vi "WiFi lab coordinator API.vi"() -> ()   [LabVIEW 2021]
uses:
  WiFi API Frame Type.ctl
  WiFi API Frame.ctl
  stop button.vi
  <vilib>/Utility/file.llb/Write Delimited Spreadsheet (string).vi
panel:
  in  "Response TCP":string
  in  "stop":bool
  in  "Response UDP":string
  in  "Control string":string
  in  "Start session":bool
  in  "Destination port (hex)":u16=9750 step=1 format="%04x"
  in  "Source port (hex)":u16=2000 step=1 format="%04x"
  out "IPs":T1(array[cluster])
  out "Payload":string
  out "Frame Type":T2 items=["Frame Error"=254, "Device Response Status"=186, "Device Request"=185, "Send Data Response"=184, "RX Packet IPv4"=176, "Zigbee Remote AT Command Response"=151, "Explicit Zigbee Receive Packet"=145, "Zigbee Receive Packet"=144, "I/O Sample Rx Indicator"=143, "Zigbee TX Status"=139, "Modem Status"=138, "Transmit Status"=137, "AT Command Response"=136, "Remote Command Response"=135, "Rx Packet"=128, "Device Response"=42, "Send Data Request"=40, "TX Request IPv4"=32, "Zigbee Remote AT Command"=23, "Zigbee Explicit Transmit Packet"=17, "Zigbee Transmit Packet"=16, "AT Command "=8, "Remote AT Command Request"=7, "TX Request"=0]
  # "Session Configuration"
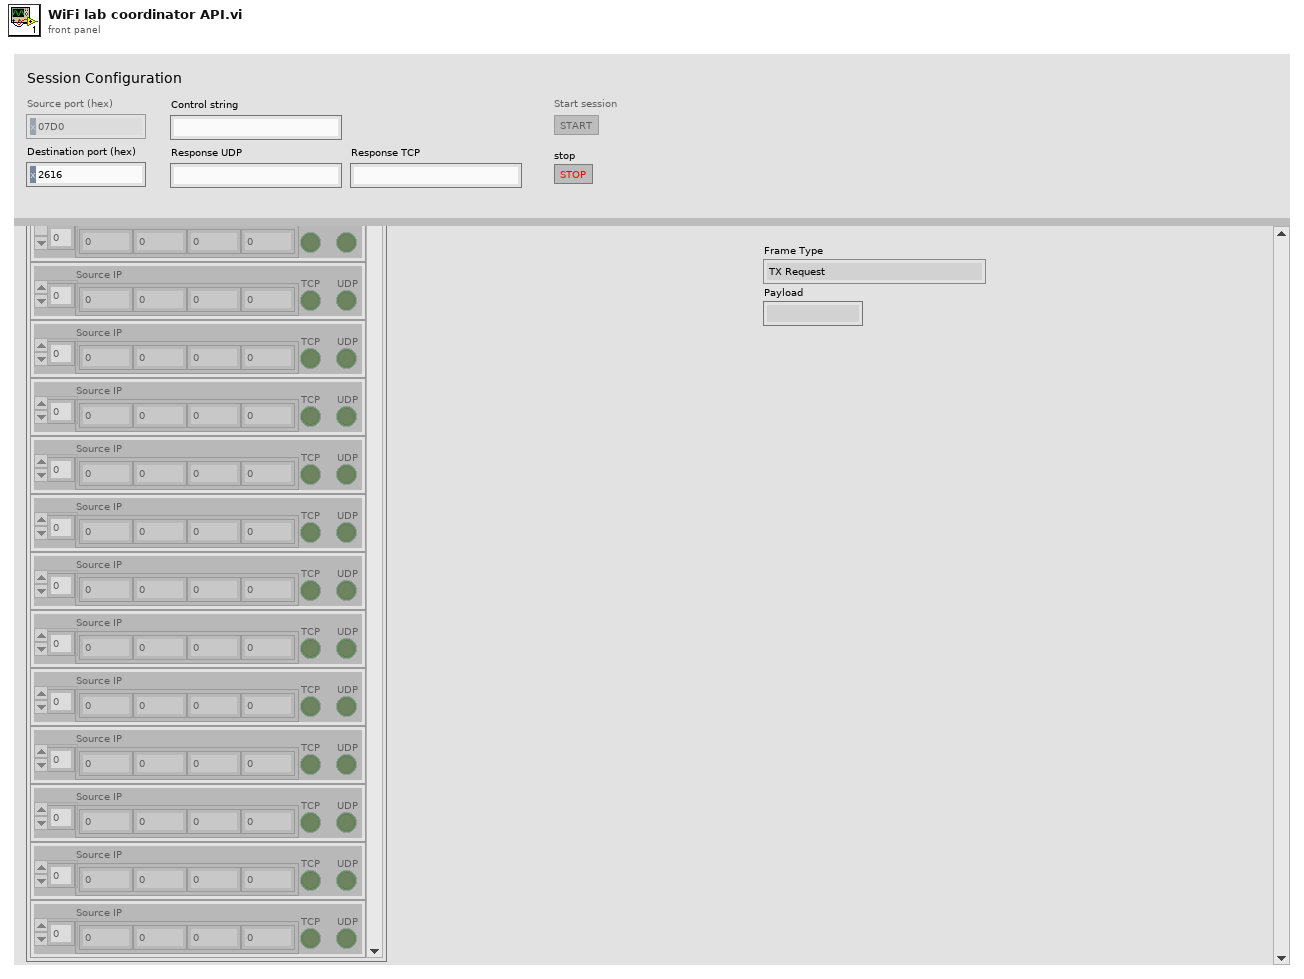
[diagram p1: front panel]
types:
  T1 = cluster{"Source IP":u8[], "TCP":bool, "UDP":bool}[]
  T2 = typedef "WiFi API Frame Type.ctl" = u8
  T3 = cluster{"Source IP":u8[], "TCP":bool, "UDP":bool}
  T4 = typedef "WiFi API Frame.ctl" = cluster{"Length":u16, "Frame Type":T2, "Payload":u8[], "Checksum":u8}
  T5 = enum8{"Enabled", "Disabled", "Disabled and Grayed Out"}
  T6 = typedef "Protocol enum.ctl" = enum8{"UDP", "TCP"}
  T7 = enum32{"invalid app kind", "Development System", "Run Time System", "Student Edition", "Embedded LabVIEW", "Evaluation", "Custom"}
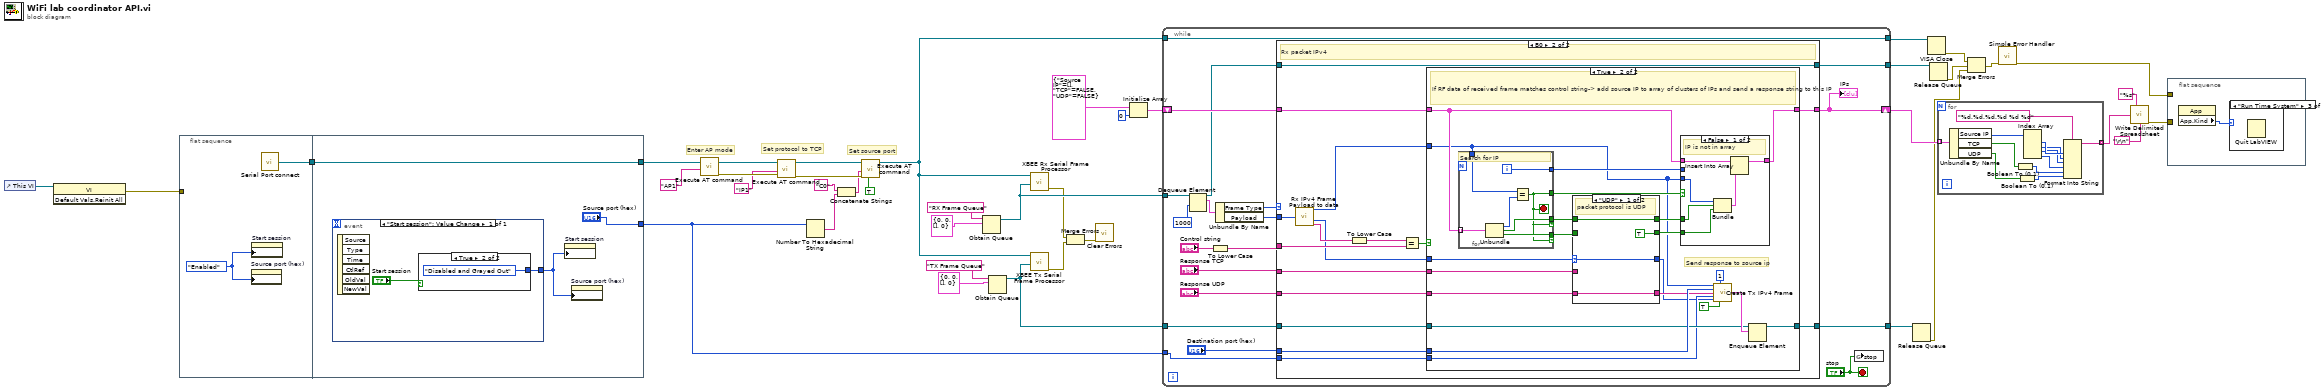
[diagram p0: block diagram]
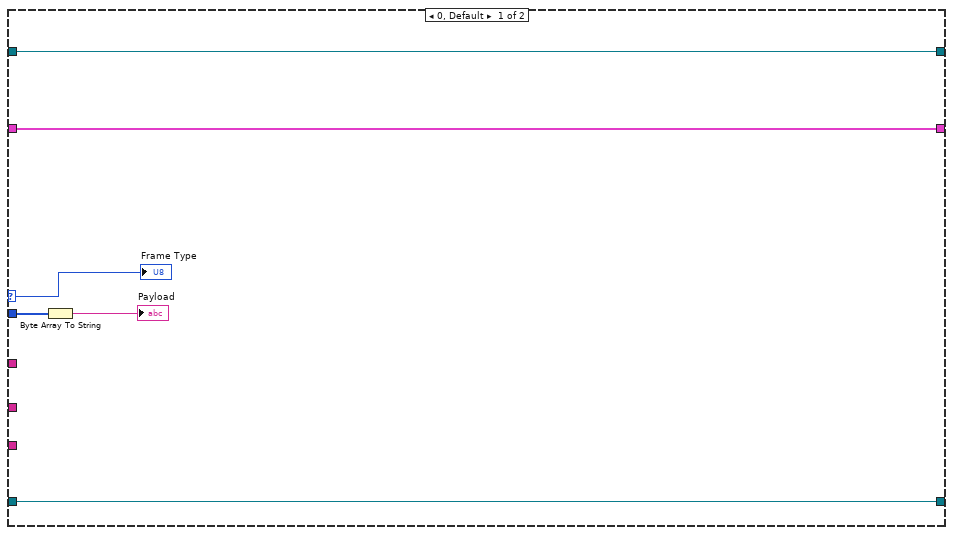
[diagram p8: hidden frame]
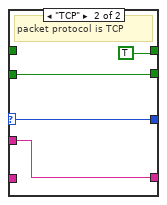
[diagram p10: hidden frame]
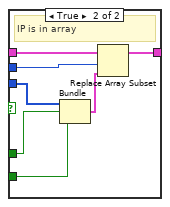
[diagram p11: hidden frame]
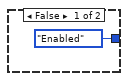
[diagram p12: hidden frame]
diagram:
  # "Set source port"
  # "Set protocol to TCP"
  # "Enter AP mode"
  n1 = control-ref of="This VI"() -> (w26:refnum<vi>)
  n2 = invoke class="VI" method="Default Vals.Reinit All"(reference=w26) -> (error out=w41:errorcluster)  [unwired: 2 in, 2 out]
  n3 = flat-sequence {
    tunnel: w41 -> [_]
    tunnel: [w42] -> w14
    tunnel: [w46] -> w27
    tunnel: w14 -> [w46]
    tunnel: ["Source port (hex)"] -> w1
    frame #0 {
      w43 = T5."Enabled" ("Disabled")
      n4 = property on="Source port (hex)" class="DigNum (strict)"("DisabledEnum"=w43) -> ()  [unwired: 2 in, 2 out]
      n5 = property on="Start session" class="Bool"("DisabledEnum"=w43) -> ()  [unwired: 2 in, 2 out]
      n6 = call "Serial Port connect.vi"() -> ("VISA resource out"=w42:refnum<visa-resource-name>)  [unwired: 1 in]
    }
    frame #1 {
      n7 = event shown="[0] \"Start session\": Value Change" {
        selector: _ -> [_]
        dyn-events: _ -> [_]
        timeout: _ -> [_]
        tunnel: [w48] -> w45
        event "Start session": Value Change {
          n8 = event-data() -> ()  [unwired: 1 in, 6 out]
          n9 = case shown="True" "Start session" {
            tunnel: [T5."Enabled" ("Disabled") T5."Disabled and Grayed Out" ("Disabled")] -> w48
            frame False {
            }
            frame True {
            }
          }
        }
      }
      n10 = property on="Start session" class="Bool"("DisabledEnum"=w45) -> ()  [unwired: 2 in, 2 out]
      n11 = property on="Source port (hex)" class="DigNum (strict)"("DisabledEnum"=w45) -> ()  [unwired: 2 in, 2 out]
    }
  }
  n12 = call "Execute AT command.vi"("AT Command"="AP1", "VISA resource in"=w27) -> ("error out"=w30:errorcluster, "VISA resource out"=w31:refnum<visa-resource-name>)  [unwired: 6 in, 1 out]
  n13 = call "Execute AT command.vi"("error in (no error)"=w30, "AT Command"="IP1", "VISA resource in"=w31) -> ("error out"=w24:errorcluster, "VISA resource out"=w25:refnum<visa-resource-name>)  [unwired: 5 in, 1 out]
  n14 = Number To Hexadecimal String(2:w1) -> (0:w20:string)  [unwired: 1 in]
  n15 = Concatenate Strings("C0" ("AT Command"), w20) -> (w21:string)
  n16 = call "Execute AT command.vi"("Exit AT mode"=TRUE, "error in (no error)"=w24, "AT Command"=w21, "VISA resource in"=w25) -> ("VISA resource out"=w23:refnum<visa-resource-name>)  [unwired: 4 in, 2 out]
  n17 = Obtain Queue(name (unnamed)="RX Frame Queue", element data type=T4 {"Length"=0, "Frame Type"=0, "Payload"=[], "Checksum"=0} ("API Frame")) -> (queue out=w36:refnum<queue>)  [unwired: 3 in, 2 out]
  n18 = Obtain Queue(name (unnamed)="TX Frame Queue", element data type=T4 {"Length"=0, "Frame Type"=0, "Payload"=[], "Checksum"=0} ("API Frame")) -> (queue out=w33:refnum<queue>)  [unwired: 3 in, 2 out]
  n19 = call "XBEE Rx Serial Frame Processor.vi"("RX Frame Queue"=w36, "VISA Serial Port"=w23) -> ("error out"=w10:errorcluster)  [unwired: 9 in]
  n20 = call "XBEE Tx Serial Frame Processor.vi"("TX Frame Queue"=w33, "VISA Serial Port"=w23) -> ("error out"=w9:errorcluster)  [unwired: 9 in]
  n21 = Merge Errors(w10, w9) -> (w11:errorcluster)
  n22 = call <vilib>:"Clear Errors.vi"("error in (no error)"=w11) -> ()  [unwired: 5 in, 2 out]
  n23 = Initialize Array(T3 {"Source IP"=[], "TCP"=FALSE, "UDP"=FALSE}, 0 ("dimension size")) -> (w35:T1)
  n24 = while {
    tunnel: w36 -> [w69]
    shift-right: [w62] -> w19
    shift-left: w35 -> [w65]
    tunnel: w33 -> [w64]
    tunnel: w23 -> [w63]
    tunnel: [w63] -> w32
    tunnel: [w54] -> w8
    tunnel: [w52] -> w7
    tunnel: w1 -> [w51]
    stop <- "stop" stop-if-true
    n25 = Dequeue Element(queue=w69, timeout in ms (-1)=1000) -> (queue out=w53:refnum<queue>, element=w68:T4)  [unwired: 1 in, 2 out]
    n26 = To Lower Case(string="Control string") -> (all lower case string=w60:string)
    n27 = Unbundle By Name(w68) -> ("Frame Type"=w67:T2, "Payload"=w66:u8[])
    n28 = case shown="B0" w67 {
      selector: w67 -> [w74 _]
      tunnel: w66 -> [w73 w91]
      tunnel: w65 -> [w75 w88]
      tunnel: w60 -> [_ w89]
      tunnel: w64 -> [w71 w90]
      tunnel: "Destination port (hex)" -> [_ w87]
      tunnel: "Response UDP" -> [_ w86]
      tunnel: w51 -> [_ w85]
      tunnel: [w75 w84] -> w62
      tunnel: "Response TCP" -> [_ w78]
      tunnel: [w71 w77] -> w54
      tunnel: w53 -> [w70 w76]
      tunnel: [w70 w76] -> w52
      frame 0, Default {
        n29 = Byte Array To String(unsigned byte array=w73) -> (string=→"Payload":string)
        "Frame Type" <- w74
      }
      frame 176 {
        # "Rx packet IPv4"
        n30 = call "Rx IPv4 Frame Payload to data.vi"("Payload array"=w91) -> ("Source IP"=w82:u8[], "Protocol"=w79:T6, "RF data"=w83:string)  [unwired: 10 in, 2 out]
        n31 = To Lower Case(string=w83) -> (all lower case string=w80:string)
        n32 = Equal?(x=w80, y=w89) -> (x = y?=w81:bool)
        n33 = case shown="True" w81 {
          tunnel: [w93 w114] -> w84
          tunnel: w90 -> [w92 w108]
          tunnel: w82 -> [_ w96]
          tunnel: w88 -> [w93 w110]
          tunnel: w87 -> [_ w109]
          tunnel: w86 -> [_ w101]
          tunnel: w85 -> [_ w106]
          tunnel: w79 -> [_ w105]
          tunnel: w78 -> [_ w99]
          tunnel: [w92 w94] -> w77
          frame False {
            # "RF data of packet does not match control string -> do nothing"
          }
          frame True {
            # "Send response to source ip"
            # "If RF data of received frame matches control string-> add source IP to array of clusters of IPs and send a response string to this IP"
            n34 = for {
              tunnel: w96 -> [w139]
              tunnel: [w136] -> w107
              tunnel: w110 -> [w142] mode=indexing
              tunnel: [w141] -> w102
              tunnel: [w138] -> w98 if=w136
              tunnel: [w137] -> w97 if=w136
              i -> [w141]
              stop <- w136 stop-if-true
              # "Search for IP"
              n35 = Unbundle(w142) -> ("Source IP"=w140:u8[], "TCP"=w138:bool, "UDP"=w137:bool)
              n36 = Equal?(x=w139, y=w140) -> (x = y?=w136:bool)
            }
            n37 = case shown="\"UDP\"" w105 {
              selector: w105 -> [w115 w119]
              tunnel: w98 -> [w118 _]
              tunnel: w97 -> [_ w121]
              tunnel: [w118 TRUE] -> w104
              tunnel: [TRUE w121] -> w103
              tunnel: w101 -> [w116 _]
              tunnel: [w116 w120] -> w100
              tunnel: w99 -> [_ w120]
              tunnel: [w115 w119] -> w95
              frame "UDP" {
                # "packet protocol is UDP"
              }
              frame "TCP" {
                # "packet protocol is TCP"
              }
            }
            n38 = case shown="False" w107 {
              tunnel: [w126 w135] -> w114
              tunnel: w110 -> [w128 w134]
              tunnel: w96 -> [w127 w133]
              tunnel: w104 -> [w124 w132]
              tunnel: w103 -> [w123 w131]
              tunnel: w102 -> [_ w129]
              frame False {
                # "IP is not in array"
                n39 = Bundle("Source IP"=w127, "TCP"=w124, "UDP"=w123) -> (w125:T3)  [unwired: 1 in]
                n40 = Insert Into Array(array=w128, new element=w125) -> (w126:T1)  [unwired: 1 in]
              }
              frame True {
                # "IP is in array"
                n41 = Bundle("Source IP"=w133, "TCP"=w132, "UDP"=w131) -> (w130:T3)  [unwired: 1 in]
                n42 = Replace Array Subset(array=w134, new element=w130, index=w129) -> (w135:T1)
              }
            }
            n43 = call "Create Tx IPv4 Frame.vi"("Destination IP"=w96, "Frame ID"=u8 1, "Destination port"=w109, "RF data"=w100, "Source port"=w106, "Protocol"=w95, "Transmit options bitfield"=TRUE) -> ("TX IPv4 Frame"=w111:T4)  [unwired: 8 in]
            n44 = Enqueue Element(queue=w108, element=w111) -> (queue out=w94:refnum<queue>)  [unwired: 2 in, 2 out]
          }
        }
      }
    }
    "IPs" <- w62
    n45 = global write "stop button.vi" "stop"("stop") -> ()
  }
  n46 = Release Queue(queue=w8) -> (error out=w2:errorcluster)  [unwired: 2 in, 2 out]
  n47 = VISA Close(VISA resource name=w32) -> (error out=w6:errorcluster)  [unwired: 1 in]
  n48 = Release Queue(queue=w7) -> (error out=w5:errorcluster)  [unwired: 2 in, 2 out]
  n49 = for {
    tunnel: w19 -> [w154] mode=indexing
    tunnel: [w143] -> w17 mode=indexing
    n50 = Unbundle By Name(w154) -> ("Source IP"=w152:u8[], "TCP"=w147:bool, "UDP"=w144:bool)
    n51 = Boolean To (0,1)(Boolean=w147) -> (0, 1=w146:i16)
    n52 = Boolean To (0,1)(Boolean=w144) -> (0, 1=w145:i16)
    n53 = Index Array(array=w152) -> (element #1=w151:u8, element #2=w150:u8, element #3=w149:u8, element #4=w148:u8)  [unwired: 4 in]
    n54 = Format Into String(format string="%d.%d.%d.%d %d %d", w151, w150, w149, w148, w146, w145) -> (resulting string=w143:string)  [unwired: 2 in, 1 out]
  }
  n55 = Merge Errors(w6, w5, w2) -> (w4:errorcluster)
  n56 = call <vilib>:"Simple Error Handler.vi"("error in (no error)"=w4) -> ("error out"=w3:errorcluster)  [unwired: 4 in, 4 out]
  n57 = call-poly <vilib>:"Write Delimited Spreadsheet.vi"("format (%s)"="%s" ("format (%.3f)"), "1D data"=w17, "delimiter (\\t)"="\r\n") -> ("error out"=w15:errorcluster)  [unwired: 11 in, 1 out]
  n58 = flat-sequence {
    tunnel: w15 -> [_]
    tunnel: w3 -> [_]
    frame #0 {
      n59 = property class="App"() -> ("App.Kind"=w155:T7)  [unwired: 2 in, 2 out]
      n60 = case shown="\"Run Time System\"" w155 {
        frame "invalid app kind", Default {
        }
        frame "Development System" {
        }
        frame "Run Time System" {
          n61 = Quit LabVIEW() -> ()  [unwired: 1 in]
        }
        frame "Student Edition" {
        }
        frame "Embedded LabVIEW" {
        }
        frame "Evaluation" {
        }
        frame "Custom" {
        }
      }
    }
  }
